vi "黑盾命令发送组合.vi"(7 "参数":u16=3000, 9 "设定参数（定点数）选择":T1(ring), 10 "遥控参数选择":T2(ring), 11 "CID2枚举":T3(ring)) -> (3 "连接的字符串":string)   [LabVIEW 2016, in "环境动力监测库.lvlib" / "空调库.lvlib"]
panel:
  in  "ADR":u8=1 format="%xH"
  in  "SOI":u8=126 format="%xH"
  in  "EOI":u16=13 format="%xH"
  out "INFO":u8 format="%xH"
  out "LENGTH":u8 format="%xH"
  out "CID2":u8 format="%xH"
  in  "CID1":u8=96 format="%xH"
  in  "VER":u8=32 format="%xH"
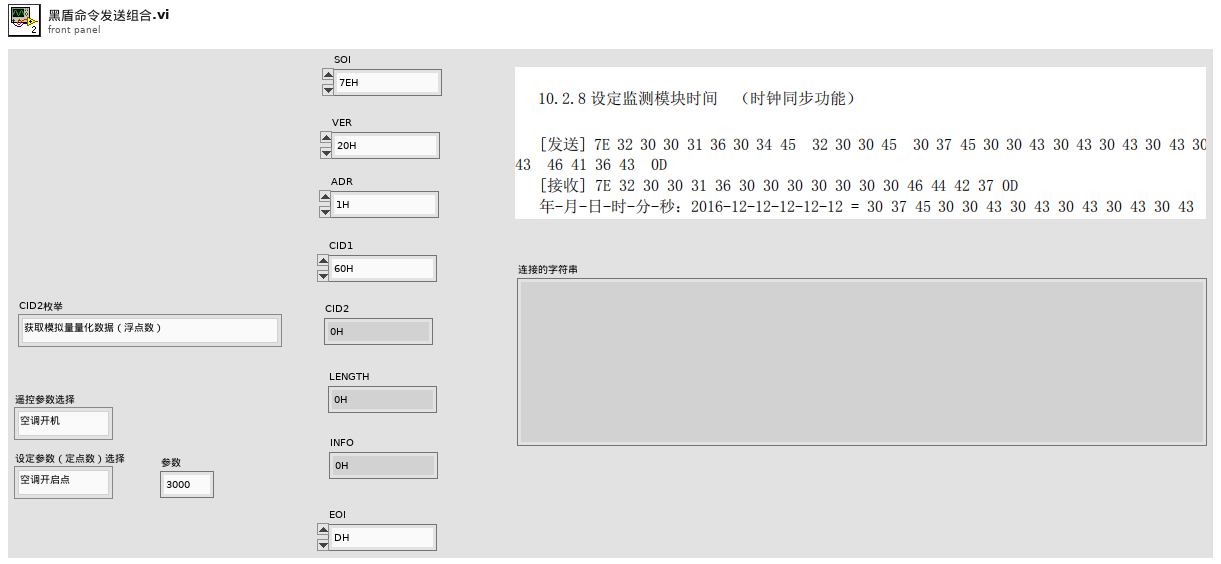
[diagram p1: front panel]
types:
  T1 = enum16{"空调开启点", "空调灵敏点", "加热开启点", "加热灵敏度", "高温告警点", "低温告警点"}
  T2 = enum16{"空调开机", "空调关机", "制冷开启", "制冷关闭", "制热开启", "制热关闭"}
  T3 = enum16{"获取模拟量量化数据（浮点数）", "获取模拟量量化数据（定点数）", "获取开关输入状态", "获取机柜空调告警状态", "遥控", "获取系统参数（浮点数）", "获取系统参数（定点数）", "设定系统参数（浮点数）", "设定系统参数（定点数）", "获取系统历史数据（浮点数）", "获取系统历史数据（定点数）", "获取历史告警", "获取监测模块时间", "设定监测模块时间", "获取通信协议版本号", "获取设备地址", "获取设备厂家信息", "设定设备地址（ADR）"}
  T4 = typedef "LVDateTimeRec.ctl" = cluster{"秒数的小数部分":dbl, "秒":i32, "分":i32, "时":i32, "日":i32, "月":i32, "年":i32, "天数（周）":i32, "天数（年）":i32, "DST":i32}
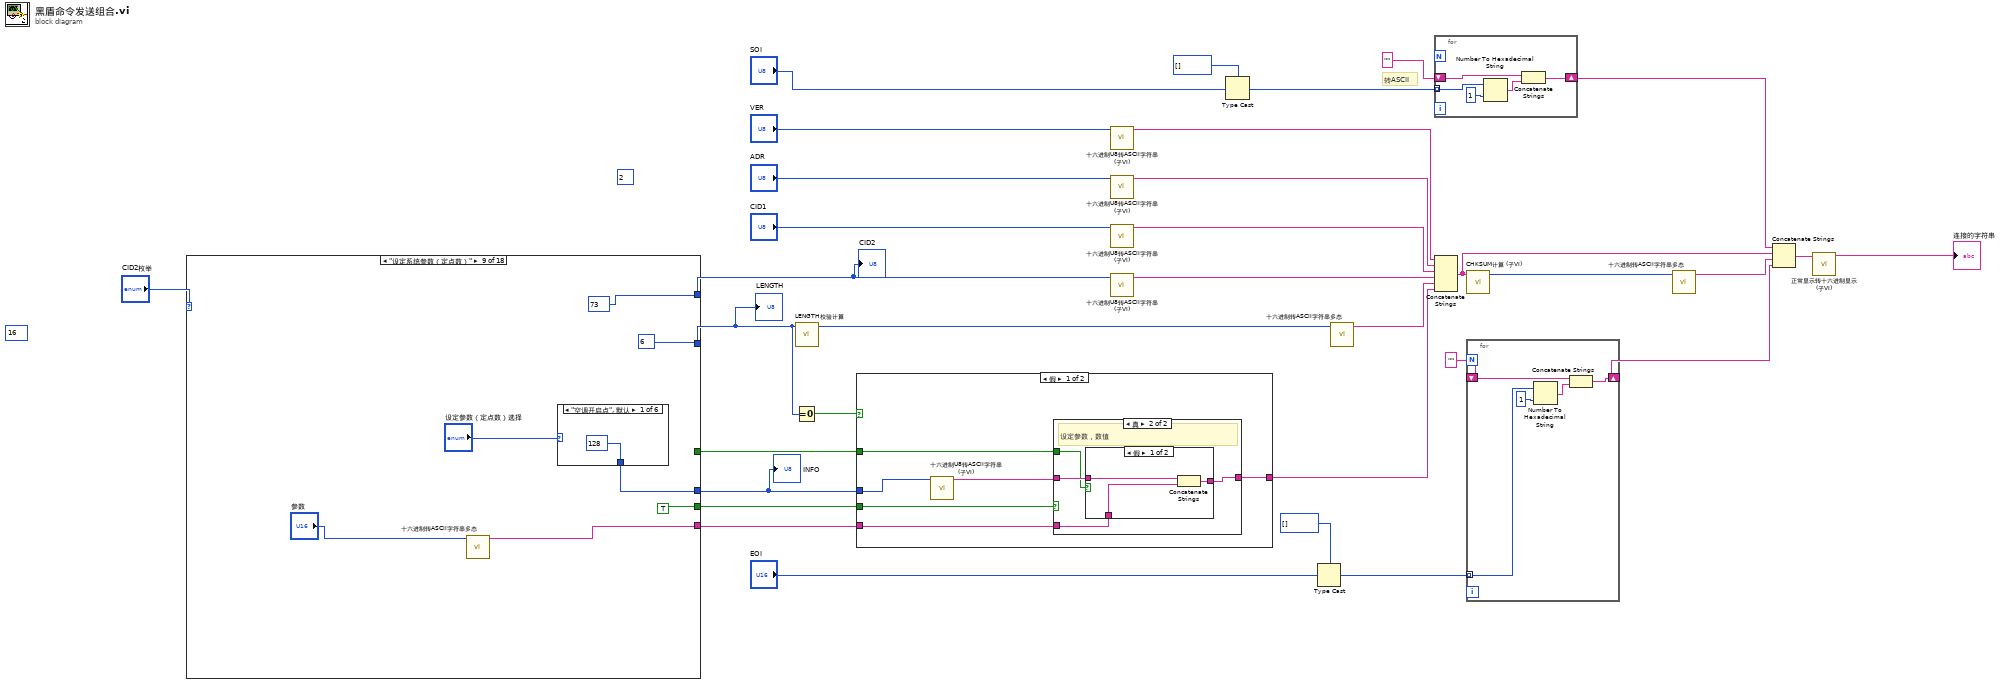
[diagram p0: block diagram]
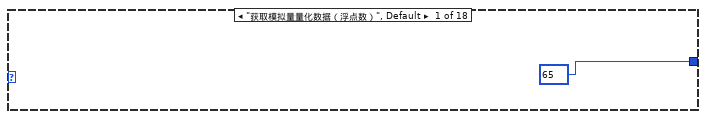
[diagram p2: hidden frame]
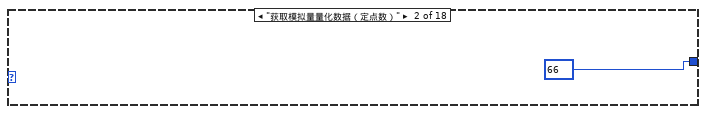
[diagram p3: hidden frame]
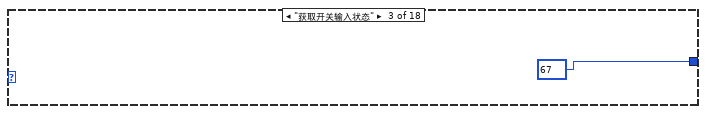
[diagram p4: hidden frame]
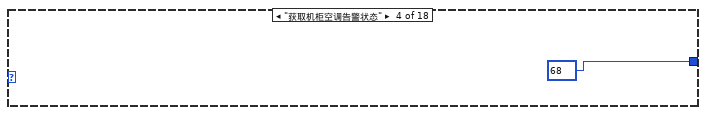
[diagram p5: hidden frame]
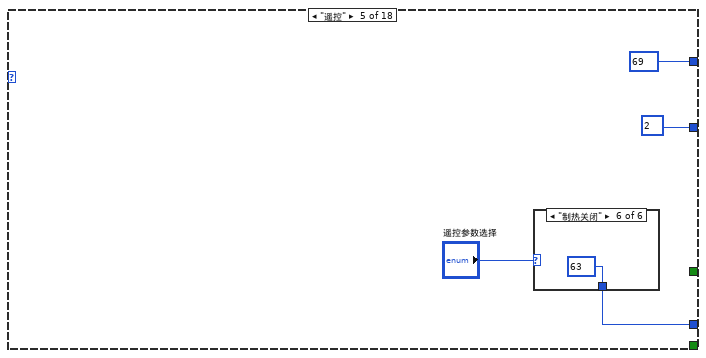
[diagram p6: hidden frame]
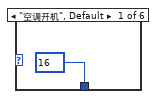
[diagram p7: hidden frame]
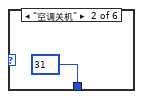
[diagram p8: hidden frame]
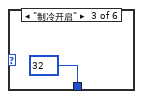
[diagram p9: hidden frame]
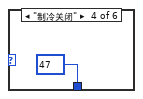
[diagram p10: hidden frame]
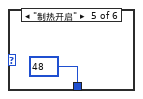
[diagram p11: hidden frame]
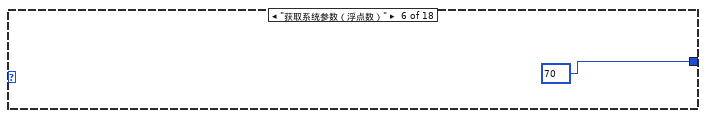
[diagram p12: hidden frame]
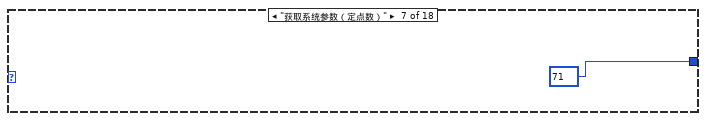
[diagram p13: hidden frame]
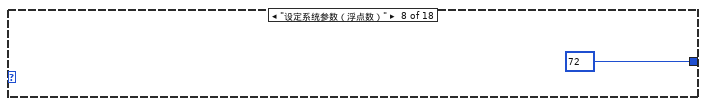
[diagram p14: hidden frame]
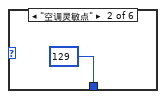
[diagram p15: hidden frame]
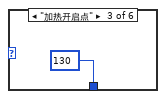
[diagram p16: hidden frame]
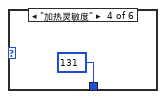
[diagram p17: hidden frame]
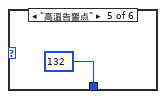
[diagram p18: hidden frame]
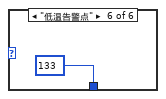
[diagram p19: hidden frame]
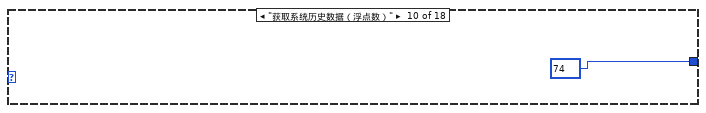
[diagram p20: hidden frame]
diagram:
  (unwired) u8 2 ("CID2")
  (unwired) u8 16 ("CID2")
  # "转ASCII"
  n1 = case shown="\"设定系统参数（定点数）\"" "CID2枚举" {
    tunnel: [u8 65 ("CID2") u8 66 ("CID2") u8 67 ("CID2") u8 68 ("CID2") u8 69 ("CID2") u8 70 ("CID2") u8 71 ("CID2") u8 72 ("CID2") u8 73 ("CID2") u8 74 ("CID2") u8 75 ("CID2") u8 76 ("CID2") u8 77 ("CID2") u8 78 ("CID2") u8 79 ("CID2") u8 80 ("CID2") u8 81 ("CID2") u8 128 ("CID2")] -> w8
    tunnel: [_ _ _ _ w39 _ _ _ w54 _ _ _ _ _ _ _ _ _] -> w7
    tunnel: [_ _ _ _ u8 2 ("CID2") _ _ _ u8 6 ("CID2") _ _ _ _ u8 14 ("CID2") _ _ _ _] -> w6
    tunnel: [_ _ _ _ _ _ _ _ TRUE _ _ _ _ TRUE _ _ _ _] -> w5
    tunnel: [_ _ _ _ _ _ _ _ w52 _ _ _ _ w70 _ _ _ _] -> w4
    tunnel: [_ _ _ _ _ _ _ _ _ _ _ _ _ TRUE _ _ _ _] -> w1
    frame "获取模拟量量化数据（浮点数）", Default {
    }
    frame "获取模拟量量化数据（定点数）" {
    }
    frame "获取开关输入状态" {
    }
    frame "获取机柜空调告警状态" {
    }
    frame "遥控" {
      n2 = case shown="\"制热关闭\"" "遥控参数选择" {
        tunnel: [u8 16 ("CID2") u8 31 ("CID2") u8 32 ("CID2") u8 47 ("CID2") u8 48 ("CID2") u8 63 ("CID2")] -> w39
        frame "空调开机", Default {
        }
        frame "空调关机" {
        }
        frame "制冷开启" {
        }
        frame "制冷关闭" {
        }
        frame "制热开启" {
        }
        frame "制热关闭" {
        }
      }
    }
    frame "获取系统参数（浮点数）" {
    }
    frame "获取系统参数（定点数）" {
    }
    frame "设定系统参数（浮点数）" {
    }
    frame "设定系统参数（定点数）" {
      n3 = call-poly "十六进制转ASCII字符串多态.vi"("十六进制数值"="参数") -> ("ASCII字符串输出"=w52:string)  [unwired: 10 in]
      n4 = case shown="\"空调开启点\", 默认" "设定参数（定点数）选择" {
        tunnel: [u8 128 ("CID2") u8 129 ("CID2") u8 130 ("CID2") u8 131 ("CID2") u8 132 ("CID2") u8 133 ("CID2")] -> w54
        frame "空调开启点", Default {
        }
        frame "空调灵敏点" {
        }
        frame "加热开启点" {
        }
        frame "加热灵敏度" {
        }
        frame "高温告警点" {
        }
        frame "低温告警点" {
        }
      }
    }
    frame "获取系统历史数据（浮点数）" {
    }
    frame "获取系统历史数据（定点数）" {
    }
    frame "获取历史告警" {
    }
    frame "获取监测模块时间" {
    }
    frame "设定监测模块时间" {
      n5 = Get Date/Time In Seconds() -> (seconds since 1Jan1904=w71:timestamp)
      n6 = Seconds To Date/Time(time stamp (now)=w71) -> (date time rec=w72:T4)  [unwired: 1 in]
      n7 = Unbundle By Name(w72) -> ("年"=w78:i32, "月"=w77:i32, "日"=w76:i32, "时"=w75:i32, "分"=w74:i32, "秒"=w73:i32)
      n8 = call-poly "十六进制转ASCII字符串多态.vi"("十六进制数值"=w75) -> ("ASCII字符串输出"=w82:string)  [unwired: 10 in]
      n9 = call-poly "十六进制转ASCII字符串多态.vi"("十六进制数值"=w73) -> ("ASCII字符串输出"=w84:string)  [unwired: 10 in]
      n10 = call-poly "十六进制转ASCII字符串多态.vi"("十六进制数值"=w76) -> ("ASCII字符串输出"=w81:string)  [unwired: 10 in]
      n11 = call-poly "十六进制转ASCII字符串多态.vi"("十六进制数值"=w74) -> ("ASCII字符串输出"=w83:string)  [unwired: 10 in]
      n12 = call-poly "十六进制转ASCII字符串多态.vi"("十六进制数值"=w77) -> ("ASCII字符串输出"=w80:string)  [unwired: 10 in]
      n13 = call-poly "十六进制转ASCII字符串多态.vi"("十六进制数值"=w78) -> ("ASCII字符串输出"=w79:string)  [unwired: 10 in]
      n14 = Concatenate Strings(w79, w80, w81, w82, w83, w84) -> (w70:string)
    }
    frame "获取通信协议版本号" {
    }
    frame "获取设备地址" {
    }
    frame "获取设备厂家信息" {
    }
    frame "设定设备地址（ADR）" {
    }
  }
  "CID2" <- w8
  "LENGTH" <- w6
  "INFO" <- w7
  n15 = Equal To 0?(x=w6) -> (x = 0?=w29:bool)
  n16 = call "LENGTH校验计算.vi"("info字节数"=w6) -> ("LENGTH"=w11:u16)  [unwired: 10 in]
  n17 = case shown="假" w29 {
    tunnel: [w94 ""] -> w28
    tunnel: w7 -> [w96 _]
    tunnel: w5 -> [w93 _]
    tunnel: w4 -> [w92 _]
    tunnel: w1 -> [w91 _]
    frame False {
      n18 = call "十六进制U8转ASCII字符串 (子VI).vi"("十六进制数值"=w96) -> ("ASCII字符串输出"=w95:string)  [unwired: 10 in]
      n19 = case shown="真" w93 {
        tunnel: w95 -> [w97 w101]
        tunnel: [w97 w100] -> w94
        tunnel: w92 -> [_ w99]
        tunnel: w91 -> [_ w98]
        frame False {
        }
        frame True {
          # "设定参数，数值"
          n20 = case shown="假" w98 {
            tunnel: w101 -> [w104 _]
            tunnel: [w103 w105] -> w100
            tunnel: w99 -> [w102 w105]
            frame False {
              n21 = Concatenate Strings(w104, w102) -> (w103:string)
            }
            frame True {
              # "设定系统时间"
            }
          }
        }
      }
    }
    frame True {
    }
  }
  n22 = call "十六进制U8转ASCII字符串 (子VI).vi"("十六进制数值"="VER") -> ("ASCII字符串输出"=w14:string)  [unwired: 10 in]
  n23 = call "十六进制U8转ASCII字符串 (子VI).vi"("十六进制数值"="ADR") -> ("ASCII字符串输出"=w15:string)  [unwired: 10 in]
  n24 = call "十六进制U8转ASCII字符串 (子VI).vi"("十六进制数值"="CID1") -> ("ASCII字符串输出"=w21:string)  [unwired: 10 in]
  n25 = call "十六进制U8转ASCII字符串 (子VI).vi"("十六进制数值"=w8) -> ("ASCII字符串输出"=w22:string)  [unwired: 10 in]
  n26 = Type Cast(type=u8[] [] ("无符号字节数组 2"), x="SOI") -> (*(type *) &x=w32:u8[])
  n27 = Type Cast(type=u8[] [] ("无符号字节数组 2"), x="EOI") -> (*(type *) &x=w19:u8[])
  n28 = call-poly "十六进制转ASCII字符串多态.vi"("十六进制数值"=w11) -> ("ASCII字符串输出"=w10:string)  [unwired: 10 in]
  n29 = for {
    tunnel: w32 -> [w111] mode=indexing
    shift-right: [w108] -> w27
    shift-left: "" -> [w109]
    n30 = Number To Hexadecimal String(1:i16 1 ("宽度(-)"), 2:w111) -> (0:w107:string)
    n31 = Concatenate Strings(w109, w107) -> (w108:string)
  }
  n32 = Concatenate Strings(w14, w15, w21, w22, w10, w28) -> (w26:string)
  n33 = call "CHKSUM计算 (子VI).vi"("发送ASCII字符"=w26) -> ("CHECKSUM"=w13:u16)  [unwired: 10 in]
  n34 = for {
    tunnel: w19 -> [w116] mode=indexing
    shift-right: [w113] -> w16
    shift-left: "" -> [w114]
    n35 = Number To Hexadecimal String(1:i16 1 ("宽度(-)"), 2:w116) -> (0:w112:string)
    n36 = Concatenate Strings(w114, w112) -> (w113:string)
  }
  n37 = call-poly "十六进制转ASCII字符串多态.vi"("十六进制数值"=w13) -> ("ASCII字符串输出"=w12:string)  [unwired: 10 in]
  n38 = Concatenate Strings(w27, w26, w12, w16) -> (w3:string)
  n39 = call "正常显示转十六进制显示 (子VI).vi"("字符串输入"=w3) -> ("字符串输出"=→"连接的字符串":string)  [unwired: 10 in]
